vi "gold--constant.vi"() -> (1 "Gold":u32(colorbox))   [LabVIEW 2018]
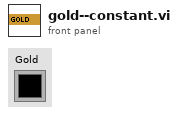
[diagram p1: front panel]
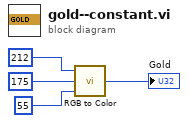
[diagram p0: block diagram]
diagram:
  n1 = call <vilib>:"RGB to Color.vi"("B"=u8 55, "G"=u8 175, "R"=u8 212) -> ("Color"=→"Gold":u32)
